vi "Filter Correction No Objects.vi"(10 "Read Power":dbl, 11 "Cluster In":T2={"Wavelength"=0.0, "AVG"=0, "Range"=0, "Backlight"=0, "Beeper"=0, "Zero"=0, "Local Lockout"=0, "ATTN"=0, "Run/Stop"=0, "Units"=0, "Averaging Points"=0, "Averaging"=FALSE, "Most Recent Power"=5.5, "Filter"=1} {"AVG" items=["Slow"=1, "Medium"=2, "Fast"=3]; "Range" items=["Auto", "Lowest", "2", "3", "4", "5", "6", "7", "Highest"]; "Backlight" items=["Off", "Low", "High"]; "Beeper" items=["Off", "On"]; "Zero" items=["Off", "On"]; "Local Lockout" items=["Off", "On"]; "ATTN" items=["Off", "On"]; "Run/Stop" items=["Stop", "Run"]; "Units" items=["W"=1, "dB"=2, "dBm"=3, "REL"=4]; "Filter" items=["Orange"=1, "Green"=2, "Yellow"=3]}) -> (2 "Corrected Power":dbl, 3 "Cluster Out":T2={"Wavelength"=0.0, "AVG"=0, "Range"=0, "Backlight"=0, "Beeper"=0, "Zero"=0, "Local Lockout"=0, "ATTN"=0, "Run/Stop"=0, "Units"=0, "Averaging Points"=0, "Averaging"=FALSE, "Most Recent Power"=5.5, "Filter"=1} {"AVG" items=["Slow"=1, "Medium"=2, "Fast"=3]; "Range" items=["Auto", "Lowest", "2", "3", "4", "5", "6", "7", "Highest"]; "Backlight" items=["Off", "Low", "High"]; "Beeper" items=["Off", "On"]; "Zero" items=["Off", "On"]; "Local Lockout" items=["Off", "On"]; "ATTN" items=["Off", "On"]; "Run/Stop" items=["Stop", "Run"]; "Units" items=["W"=1, "dB"=2, "dBm"=3, "REL"=4]; "Filter" items=["Orange"=1, "Green"=2, "Yellow"=3]})   [LabVIEW 2013]
doc: "Corrects the power measurement for which filter is being used."
uses:
  Public/Filters.ctl
  Newport 1830-C.lvlib
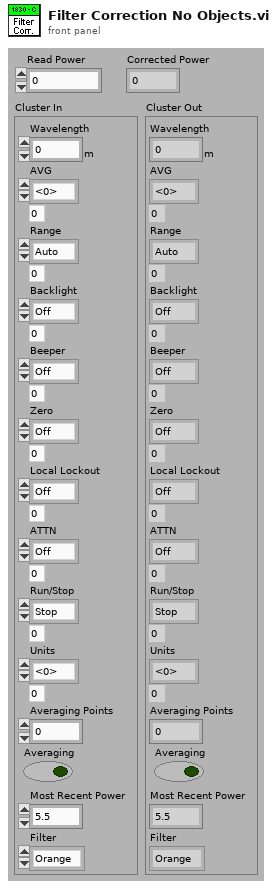
[diagram p1: front panel]
types:
  T1 = typedef "Newport 1830-C.lvlib/Filters.ctl" = u16
  T2 = cluster{"Wavelength":dbl[unit], "AVG":u16, "Range":u16, "Backlight":u16, "Beeper":u16, "Zero":u16, "Local Lockout":u16, "ATTN":u16, "Run/Stop":u16, "Units":u16, "Averaging Points":u32, "Averaging":bool, "Most Recent Power":dbl, "Filter":T1}
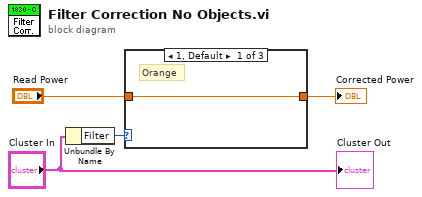
[diagram p0: block diagram]
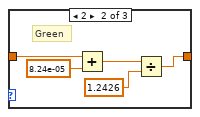
[diagram p2: hidden frame]
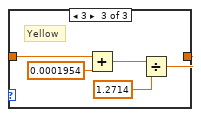
[diagram p3: hidden frame]
diagram:
  n1 = Unbundle By Name("Cluster In") -> ("Filter"=w4:T1)
  n2 = case shown="1, Default" w4 {
    tunnel: "Read Power" -> [w5 w7 w12]
    tunnel: [w5 w6 w11] -> w3
    frame 1, Default {
      # "Orange"
    }
    frame 2 {
      # "Green"
      n3 = Add(x=w7, y=8.24e-05) -> (x+y=w8:dbl)
      n4 = Divide(x=w8, y=1.2426) -> (x/y=w6:dbl)
    }
    frame 3 {
      # "Yellow"
      n5 = Add(x=w12, y=0.0001954) -> (x+y=w13:dbl)
      n6 = Divide(x=w13, y=1.2714) -> (x/y=w11:dbl)
    }
  }
  "Corrected Power" <- w3
  "Cluster Out" <- "Cluster In"
